vi "mainVI_SIL.vi"(5 "Supervisor in":refnum<class "Supervisor.lvclass">, 7 "Vessel in":refnum<class "Vessel.lvclass">, 8 "error out":errorcluster, 9 "NAVI string":string="!init;50;70;0;0;;;;", 10 "ROV string":string="34.5,,,,$56.3,34.556,,,,$67.9", 11 "Iteration Number":i32) -> (0 "error out 2":errorcluster, 1 "Cancel Button":bool, 2 "telebuf":u8[](array[numeric]), 4 "Supervisor out":refnum<class "Supervisor.lvclass">, 6 "Vessel out":refnum<class "Vessel.lvclass">)   [LabVIEW 2011]
doc: "The main VI"
uses:
  Supervisor/Supervisor.lvclass
  ROV/Vessel.lvclass
panel:
  in  "MT_DATA":sgl[](array[numeric])=[0.0, 0.0, 0.0, 0.0, 0.0, 0.0, 0.0, 0.0, 0.0, 0.0, 0.0, 0.0]
  in  "MRU out":dbl[](array[numeric])=[0.0, 0.0, 0.0, 0.0, 0.0, 0.0, 0.0, 0.0]
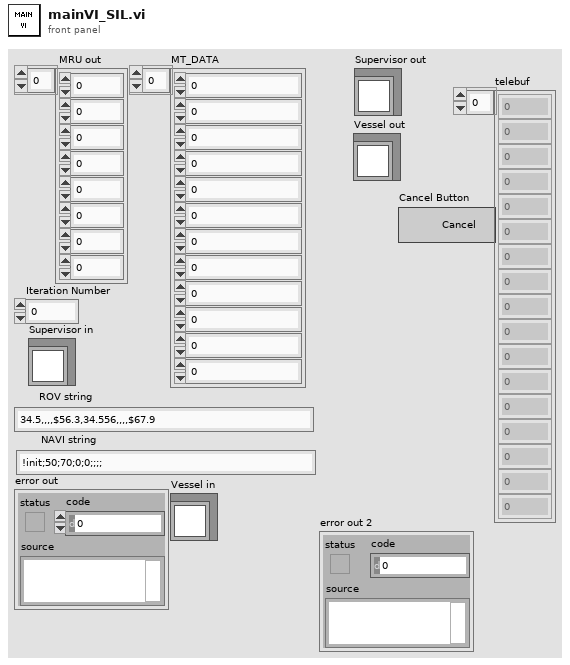
[diagram p1: front panel]
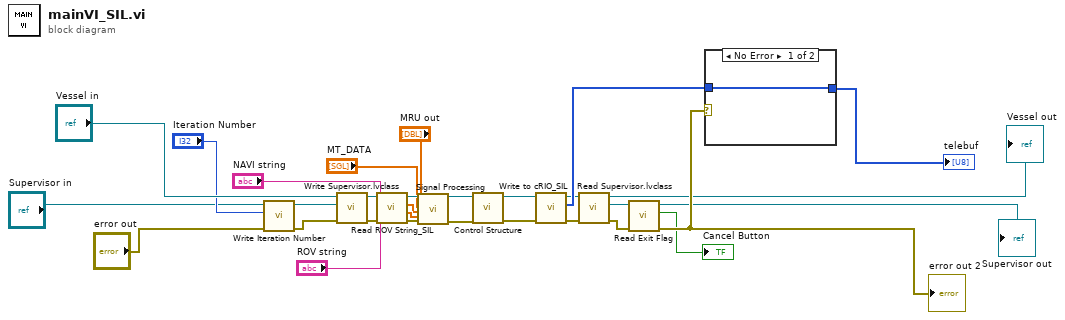
[diagram p0: block diagram]
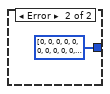
[diagram p2: hidden frame]
diagram:
  n1 = call-dynamic "Write Iteration Number.vi"("error in (no error)"="error out", "Iteration Number"="Iteration Number", "Supervisor in"="Supervisor in") -> ("error out"=w20:errorcluster, "Supervisor out"=w21:refnum<class "Supervisor.lvclass">)  [unwired: 7 in]
  n2 = call "Write Supervisor.lvclass.vi"("error in (no error)"=w20, "Supervisor.lvclass"=w21, "Vessel in"="Vessel in") -> ("error out"=w13:errorcluster, "Vessel out"=w14:refnum<class "Vessel.lvclass">)  [unwired: 7 in]
  n3 = call-dynamic "Read ROV String_SIL.vi"("error in (no error)"=w13, "NAVI string"="NAVI string", "ROV string"="ROV string", "Vessel in"=w14) -> ("error out"=w12:errorcluster, "dvl_m"=w11:dbl[], "Signals out"=w10:dbl[], "Vessel out"=w15:refnum<class "Vessel.lvclass">)  [unwired: 4 in]
  n4 = call-dynamic "Signal Processing.vi"("Vessel in"=w15, "MRU out"="MRU out", "MT_DATA"="MT_DATA", "Signals in"=w10, "dvl_m"=w11, "error in (no error)"=w12) -> ("Vessel out"=w23:refnum<class "Vessel.lvclass">, "error out"=w22:errorcluster)  [unwired: 12 in]
  n5 = call "Control Structure.vi"("error in (no error)"=w22, "Vessel in"=w23) -> ("error out"=w18:errorcluster, "Vessel out"=w19:refnum<class "Vessel.lvclass">)  [unwired: 8 in]
  n6 = call-dynamic "Write to cRIO_SIL.vi"("error in (no error)"=w18, "Vessel in"=w19) -> ("error out"=w16:errorcluster, "telebuf"=w25:u8[], "Vessel out"=w17:refnum<class "Vessel.lvclass">)  [unwired: 7 in]
  n7 = call "Read Supervisor.lvclass.vi"("error in (no error)"=w16, "Vessel in"=w17) -> ("error out"=w4:errorcluster, "Supervisor.lvclass"=w24:refnum<class "Supervisor.lvclass">, "Vessel out"=→"Vessel out":refnum<class "Vessel.lvclass">)  [unwired: 7 in]
  n8 = call-dynamic "Read Exit Flag.vi"("error in (no error)"=w4, "Supervisor in"=w24) -> ("error out"=w29:errorcluster, "Exit Flag"=→"Cancel Button":bool, "Supervisor out"=→"Supervisor out":refnum<class "Supervisor.lvclass">)  [unwired: 7 in]
  "error out 2" <- w29
  n9 = case shown="No Error" w29 {
    tunnel: w25 -> [w31 _]
    tunnel: [w31 u8[] [0, 0, 0, 0, 0, 0, 0, 0, 0, 0, 0, 0, 0, 0, 0, 0, 0, 0, 0] ("telebuf")] -> w30
    frame No Error {
    }
    frame Error {
    }
  }
  "telebuf" <- w30
